vi "main_runtime_display.vi"(8 "Runtime (string)":refnum<vi>, 9 "Runtime":refnum<vi>, 10 "Pause Button":refnum<vi>, 11 "Running?":refnum<vi>) -> ()   [LabVIEW 2019]
uses:
  lib/libSimulationControl/libSimulationControl.lvlib
panel:
  # "*******************************************************************\nBiogas Plant Control\n\nAuthor: Paul Zügel\nGCSC-Frankfurt am Main 2020\n\n*******************************************************************"
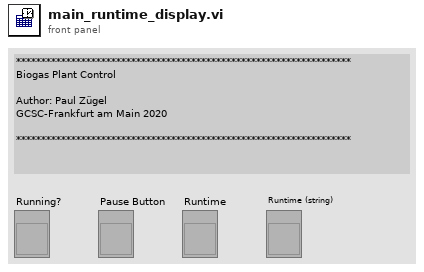
[diagram p1: front panel]
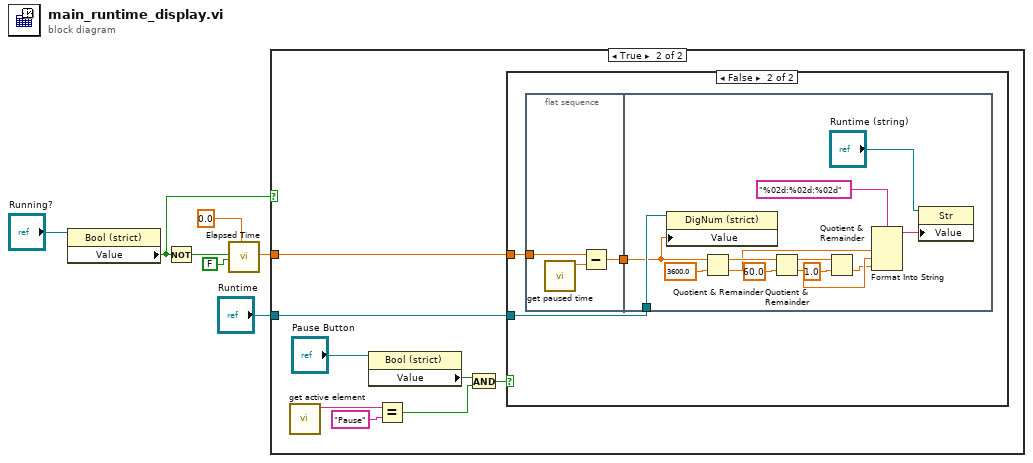
[diagram p0: block diagram]
diagram:
  n1 = property class="Bool (strict)"(reference="Running?") -> ("Value"=w7:bool)  [unwired: 1 in, 2 out]
  n2 = Not(x=w7) -> (.not. x?=w6:bool)
  n3 = call "Elapsed Time"("Reset"=w6, "Auto Reset"=FALSE, "Set Start Time (s)"=0.0) -> ("Elapsed Time (s)"=w3:dbl)  [unwired: 9 in, 7 out]
  n4 = case shown="True" w7 {
    tunnel: w3 -> [_ w10]
    tunnel: "Runtime" -> [_ w8]
    frame False {
    }
    frame True {
      n5 = call "get active element.vi"() -> ("active_element"=w14:string)  [unwired: 10 in, 1 out]
      n6 = property class="Bool (strict)"(reference="Pause Button") -> ("Value"=w13:bool)  [unwired: 1 in, 2 out]
      n7 = Equal?(x=w14, y="Pause") -> (x = y?=w12:bool)
      n8 = And(x=w13, y=w12) -> (x .and. y?=w9:bool)
      n9 = case shown="False" w9 {
        tunnel: w10 -> [_ w18]
        tunnel: w8 -> [_ w16]
        frame True {
        }
        frame False {
          n10 = flat-sequence {
            tunnel: w18 -> [w21]
            tunnel: [w20] -> w17
            tunnel: w17 -> [w24]
            tunnel: w16 -> [w34]
            frame #0 {
              n11 = call "get paused time.vi"() -> ("function return"=w19:dbl)  [unwired: 10 in, 1 out]
              n12 = Subtract(x=w21, y=w19) -> (x-y=w20:dbl)
            }
            frame #1 {
              n13 = property class="DigNum (strict)"(reference=w34, "Value"=w24) -> ()  [unwired: 1 in, 2 out]
              n14 = Quotient & Remainder(x=w24, y=3600.0) -> (x-y*floor(x/y)=w32:dbl, floor(x/y)=w28:dbl)
              n15 = Quotient & Remainder(x=w32, y=60.0) -> (x-y*floor(x/y)=w30:dbl, floor(x/y)=w27:dbl)
              n16 = Quotient & Remainder(x=w30, y=1.0) -> (floor(x/y)=w26:dbl)  [unwired: 1 out]
              n17 = Format Into String(format string="%02d:%02d:%02d" ("initial string"), w28, w27, w26) -> (resulting string=w22:string)  [unwired: 2 in, 1 out]
              n18 = property class="Str"(reference="Runtime (string)", "Value"=w22) -> ()  [unwired: 1 in, 2 out]
            }
          }
        }
      }
    }
  }
